vi "Parse Status.vi"(4 "Status":string) -> (7 "Path Statuses":T1[](array[typedef]))   [LabVIEW 2020, in "VolatusGUI.lvlib" / "Git Updater Module.lvclass"]
uses:
  Git Updater Module.lvclass
  Git Updater Module.lvclass/Git Updater Module.ctl
  Status.ctl
  Path Status.ctl
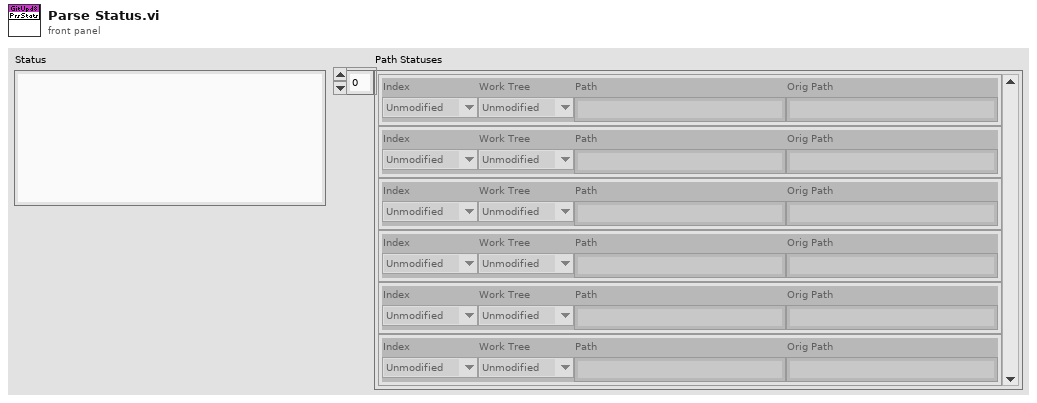
[diagram p1: front panel]
types:
  T1 = typedef "VolatusGUI.lvlib/Git Updater Module.lvclass/Path Status.ctl" = cluster{"Index":T2, "Work Tree":T2, "Path":string, "Orig Path":string}
  T2 = typedef "VolatusGUI.lvlib/Git Updater Module.lvclass/Status.ctl" = enum16{"UNKNOWN", "Unmodified", "Modified", "Added", "Deleted", "Renamed", "Unmerged", "Untracked", "Ignored"}
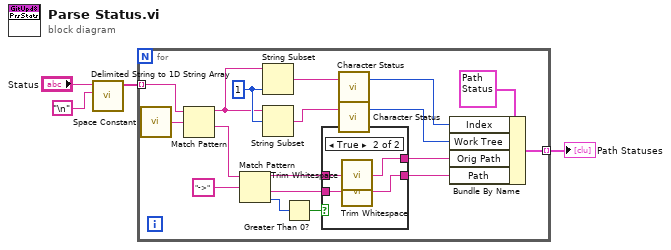
[diagram p0: block diagram]
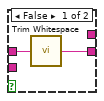
[diagram p2: hidden frame]
diagram:
  n1 = call <vilib>:"Delimited String to 1D String Array.vi"("delimiter"="\n", "delimited string"="Status") -> ("string array"=w2:string[])  [unwired: 9 in]
  n2 = for {
    tunnel: w2 -> [w22] mode=indexing
    tunnel: [w9] -> w1 mode=indexing
    w20 = 1 ("length (rest)")
    n3 = call <vilib>:"Space Constant.vi"() -> ("String"=w21:string)
    n4 = Match Pattern(string=w22, regular expression=w21) -> (before substring=w19:string, after substring=w18:string)  [unwired: 1 in, 2 out]
    n5 = Match Pattern(string=w18, regular expression="->") -> (before substring=w13:string, after substring=w14:string, offset past match=w16:i32)  [unwired: 1 in, 1 out]
    n6 = String Subset(string=w19, length (rest)=w20) -> (substring=w6:string)  [unwired: 1 in]
    n7 = String Subset(string=w19, offset (0)=w20) -> (substring=w8:string)  [unwired: 1 in]
    n8 = Greater Than 0?(x=w16) -> (x > 0?=w15:bool)
    n9 = case shown="True" w15 {
      tunnel: w14 -> [_ w27]
      tunnel: w13 -> [w24 w28]
      tunnel: [w23 w26] -> w11
      tunnel: [_ w25] -> w10
      frame False {
        n10 = call <vilib>:"Trim Whitespace.vi"("string"=w24) -> ("trimmed string"=w23:string)  [unwired: 1 in]
      }
      frame True {
        n11 = call <vilib>:"Trim Whitespace.vi"("string"=w28) -> ("trimmed string"=w25:string)  [unwired: 1 in]
        n12 = call <vilib>:"Trim Whitespace.vi"("string"=w27) -> ("trimmed string"=w26:string)  [unwired: 1 in]
      }
    }
    n13 = call "Character Status.vi"("Character"=w6) -> ("Status"=w5:T2)  [unwired: 6 in]
    n14 = call "Character Status.vi"("Character"=w8) -> ("Status"=w7:T2)  [unwired: 6 in]
    n15 = Bundle By Name(cluster=T1 {"Index"=enum."Unmodified", "Work Tree"=enum."Unmodified", "Path"="", "Orig Path"=""} ("Path Status"), "Index"=w5, "Work Tree"=w7, "Orig Path"=w10, "Path"=w11) -> (w9:T1)
  }
  "Path Statuses" <- w1
